vi "create complex multi-tone signal.vi"(6 "sampling info":cluster{"Fs":dbl, "#s":dbl}={"Fs"=1000.0, "#s"=1000.0}, 10 "Noise level":dbl=1.0, 11 "Input tones":T1(array[cluster])) -> (3 "complex waveform":waveform(cdb))   [LabVIEW 2020]
doc: "Create complex multi-tone signal."
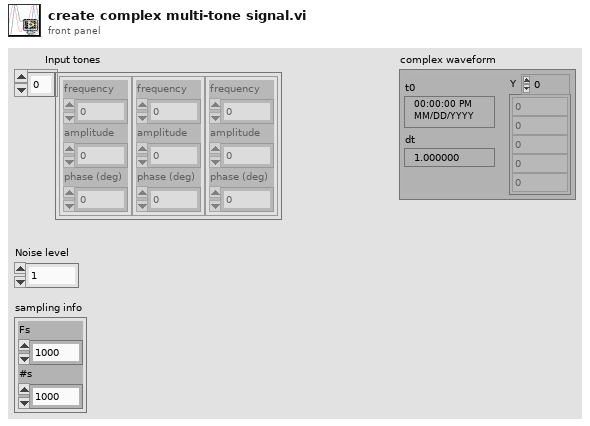
[diagram p1: front panel]
types:
  T1 = cluster{"frequency":dbl, "amplitude":dbl, "phase (deg)":dbl}[]
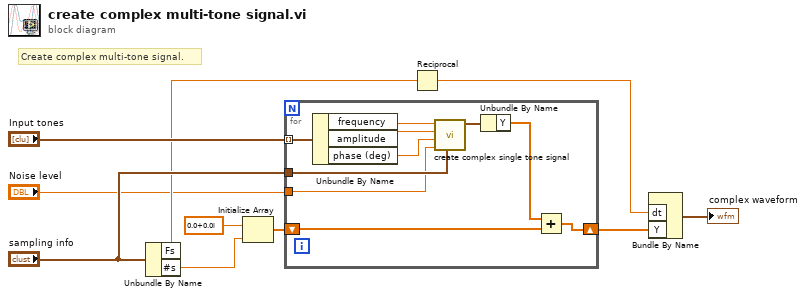
[diagram p0: block diagram]
diagram:
  # "Create complex multi-tone signal."
  n1 = Unbundle By Name("sampling info") -> ("Fs"=w4:dbl, "#s"=w3:dbl)
  n2 = Initialize Array(cdb 0.0+0.0i ("element"), w3) -> (w8:cdb[])
  n3 = for {
    tunnel: "Input tones" -> [w20] mode=indexing
    shift-right: [w14] -> w1
    shift-left: w8 -> [w15]
    tunnel: "sampling info" -> [w12]
    tunnel: "Noise level" -> [w11]
    n4 = Unbundle By Name(w20) -> ("frequency"=w19:dbl, "amplitude"=w18:dbl, "phase (deg)"=w17:dbl)
    n5 = call "create complex single tone signal.vi"("sampling info"=w12, "Noise level"=w11, "phase (deg)"=w17, "amplitude"=w18, "frequency (Hz)"=w19) -> ("complex waveform"=w16:waveform(cdb))  [unwired: 1 in, 5 out]
    n6 = Unbundle By Name(w16) -> ("Y"=w13:cdb[])
    n7 = Add(x=w13, y=w15) -> (x+y=w14:cdb[])
  }
  n8 = Reciprocal(x=w4) -> (1/x=w6:dbl)
  n9 = Bundle By Name("dt"=w6, "Y"=w1) -> (→"complex waveform":waveform(cdb))  [unwired: 1 out]
